vi "Enqueu Element.vi"(8 "Boolean":bool, 9 "Enum in":variant, 10 "Message":string, 11 "Queue in":refnum<queue>) -> (3 "queue out":refnum<queue>)   [LabVIEW 2014]
uses:
  Cntrls/Message Cluster.ctl
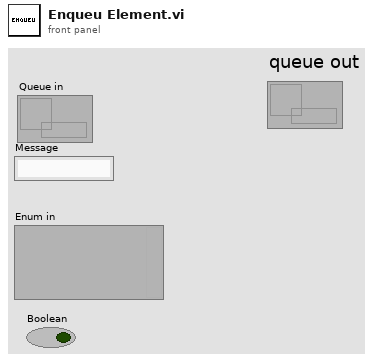
[diagram p1: front panel]
types:
  T1 = typedef "Message Cluster.ctl" = cluster{"Enum":variant, "Message":string}
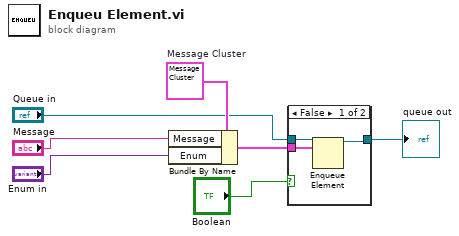
[diagram p0: block diagram]
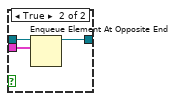
[diagram p2: hidden frame]
diagram:
  w5 = T1 {"Enum"=variant, "Message"=""}  # Message Cluster
  n1 = Bundle By Name(cluster=w5, "Message"="Message", "Enum"="Enum in") -> (w6:T1)
  n2 = case shown="False" "Boolean" {
    tunnel: w6 -> [w9 w13]
    tunnel: "Queue in" -> [w10 w12]
    tunnel: [w8 w11] -> w2
    frame False {
      n3 = Enqueue Element(queue=w10, element=w9) -> (queue out=w8:refnum<queue>)  [unwired: 2 in, 2 out]
    }
    frame True {
      n4 = Enqueue Element At Opposite End(queue=w12, element=w13) -> (queue out=w11:refnum<queue>)  [unwired: 2 in, 2 out]
    }
  }
  "queue out" <- w2
